vi "what.vi"() -> ()   [LabVIEW 2017]
uses:
  what.ctl
  <vilib>/myRIO/Instrument Drivers/Onboard IO/DIO/typedefs/DIO Reference.ctl
  <vilib>/myRIO/Common/Instrument Driver Framework/Utilities/typedefs/myRIO Generic Hardware Reference.ctl
  <vilib>/myRIO/Common/Instrument Driver Framework/Utilities/typedefs/Hardware Version Enum.ctl
  <vilib>/myRIO/Common/Instrument Driver Framework/Utilities/typedefs/myRIO v1.0 Reference.ctl
  <vilib>/myRIO/Common/Instrument Driver Framework/Utilities/typedefs/Generic FPGA Reference.ctl
  <vilib>/myRIO/Common/Instrument Driver Framework/myRIO v1.0/DIO/typedefs/DIO Channels List.ctl
  <vilib>/myRIO/Common/Instrument Driver Framework/myRIO v1.0/DIO/typedefs/DIO Channels Enum.ctl
  <vilib>/userdefined/High Color/nirio_resource_hc.ctl
  <vilib>/myRIO/Common/Instrument Driver Framework/Utilities/vis/Is FPGA Ref Available.vi
  <vilib>/myRIO/Common/Instrument Driver Framework/myRIO v1.0/DIO/vis/myRIO v1.1 Open DIO.vi
  <vilib>/myRIO/Instrument Drivers/Onboard IO/DIO/vis/Read.vi
  <vilib>/myRIO/Common/Instrument Driver Framework/Utilities/vis/Validate Channels.vi
  <vilib>/myRIO/Common/Instrument Driver Framework/myRIO v1.0/DIO/vis/myRIO v1.0 Reserve DIO.vi
  <vilib>/myRIO/Common/Instrument Driver Framework/myRIO v1.0/Resource Manager/vis/myRIO v1.0 Reserve Channel List.vi
  <vilib>/myRIO/Common/Instrument Driver Framework/myRIO v1.0/DIO/vis/myRIO v1.0 Build MUX Configuration DIO.vi
  <vilib>/myRIO/Common/Instrument Driver Framework/myRIO v1.0/Resource Manager/vis/myRIO v1.0 Reserve Channel.vi
  <vilib>/myRIO/Common/Instrument Driver Framework/myRIO v1.0/Resource Manager/vis/myRIO v1.0 Unreserve Channel.vi
  <vilib>/myRIO/Common/Instrument Driver Framework/myRIO v1.0/Resource Manager/vis/myRIO v1.0 Create Configuration List.vi
  <vilib>/myRIO/Common/Instrument Driver Framework/myRIO v1.0/Resource Manager/vis/myRIO v1.0 Build Mutex Name.vi
  <vilib>/Utility/VariantDataType/GetNumericInfo.vi
  <vilib>/Utility/error.llb/Error Cluster From Error Code.vi
  <vilib>/myRIO/Common/Instrument Driver Framework/myRIO v1.0/myRIO v1.1 Open.vi
  <vilib>/myRIO/Common/Instrument Driver Framework/Utilities/vis/IO Manager.vi
  <vilib>/myRIO/Common/Instrument Driver Framework/Utilities/vis/Configuration Manager.vi
  <vilib>/myRIO/Common/Instrument Driver Framework/myRIO v1.0/Resource Manager/vis/myRIO v1.0 Configure IO.vi
  <vilib>/myRIO/Common/Instrument Driver Framework/myRIO v1.0/myRIO v1.0 Close.vi
  <vilib>/myRIO/Common/Instrument Driver Framework/myRIO v1.0/DIO/vis/myRIO v1.0 Read DIO.vi
  <vilib>/myRIO/Express VI/Onboard IO/DI/DI Express VI.xnode
  <vilib>/myRIO/Instrument Drivers/Onboard IO/DIO/vis/myRIO DIO Open.xnode
  <vilib>/myRIO/Instrument Drivers/Onboard IO/DIO/DIO.lvlib
panel:
  out "index of element":i32
  in  "Abort":bool
  out "Counter Value":dbl
  in  "stop":bool
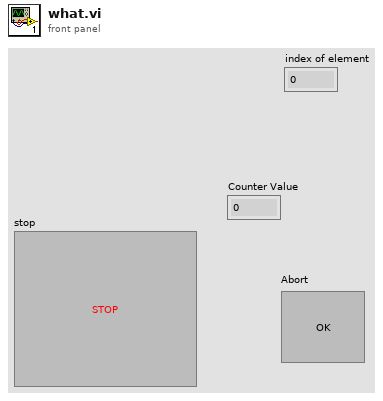
[diagram p1: front panel]
types:
  T1 = enum16{"off", "flash", "top", "middle", "bottom"}
  T2 = typedef "what.ctl" = enum16{"Initialize", "Floor 1", "Floor 2", "Floor 3", "GO!", "Stop!", "Wait for User Input"}
  T3 = typedef "DIO.lvlib/DIO Reference.ctl" = cluster{"myRIO Reference":T4, "DIO Channels List":T8}
  T4 = typedef "myRIO Generic Hardware Reference.ctl" = cluster{"myRIO Model":T5, "myRIO Hardware Reference":T6}
  T5 = typedef "Hardware Version Enum.ctl" = enum16{"Unknown", "myRIO-1900", "myRIO-1950", "roboRIO", "NI ELVIS RIO CM"}
  T6 = typedef "myRIO v1.0 Reference.ctl" = cluster{"Generic FPGA Reference":T7, "Allow multiple opens":bool}
  T7 = typedef "Generic FPGA Reference.ctl" = refnum<k20>
  T8 = typedef "DIO Channels List.ctl" = T9[]
  T9 = typedef "DIO Channels Enum.ctl" = enum16{"Not Connected", "C/DIO0", "C/DIO1", "C/DIO2", "C/DIO3", "C/DIO4", "C/DIO5", "C/DIO6", "C/DIO7", "A/DIO0", "A/DIO1", "A/DIO2", "A/DIO3", "A/DIO4", "A/DIO5", "A/DIO6", "A/DIO7", "A/DIO8", "A/DIO9", "A/DIO10", "A/DIO11", "A/DIO12", "A/DIO13", "A/DIO14", "A/DIO15", "B/DIO0", "B/DIO1", "B/DIO2", "B/DIO3", "B/DIO4", "B/DIO5", "B/DIO6", "B/DIO7", "B/DIO8", "B/DIO9", "B/DIO10", "B/DIO11", "B/DIO12", "B/DIO13", "B/DIO14", "B/DIO15", "LED0", "LED1", "LED2", "LED3", "Button0", "DIO/DIO0", "DIO/DIO1", "DIO/DIO2", "DIO/DIO3", "DIO/DIO4", "DIO/DIO5", "DIO/DIO6", "DIO/DIO7", "DIO/DIO8", "DIO/DIO9", "SPI/CS0", "SPI/CS1", "SPI/CS2", "SPI/CS3", "LED RADIO (Green)", "LED RADIO (Red)", "LED COMM (Green)", "LED COMM (Red)", "LED MODE (Green)", "LED MODE (Red)"}
  T10 = typedef "nirio_resource_hc.ctl" = tag
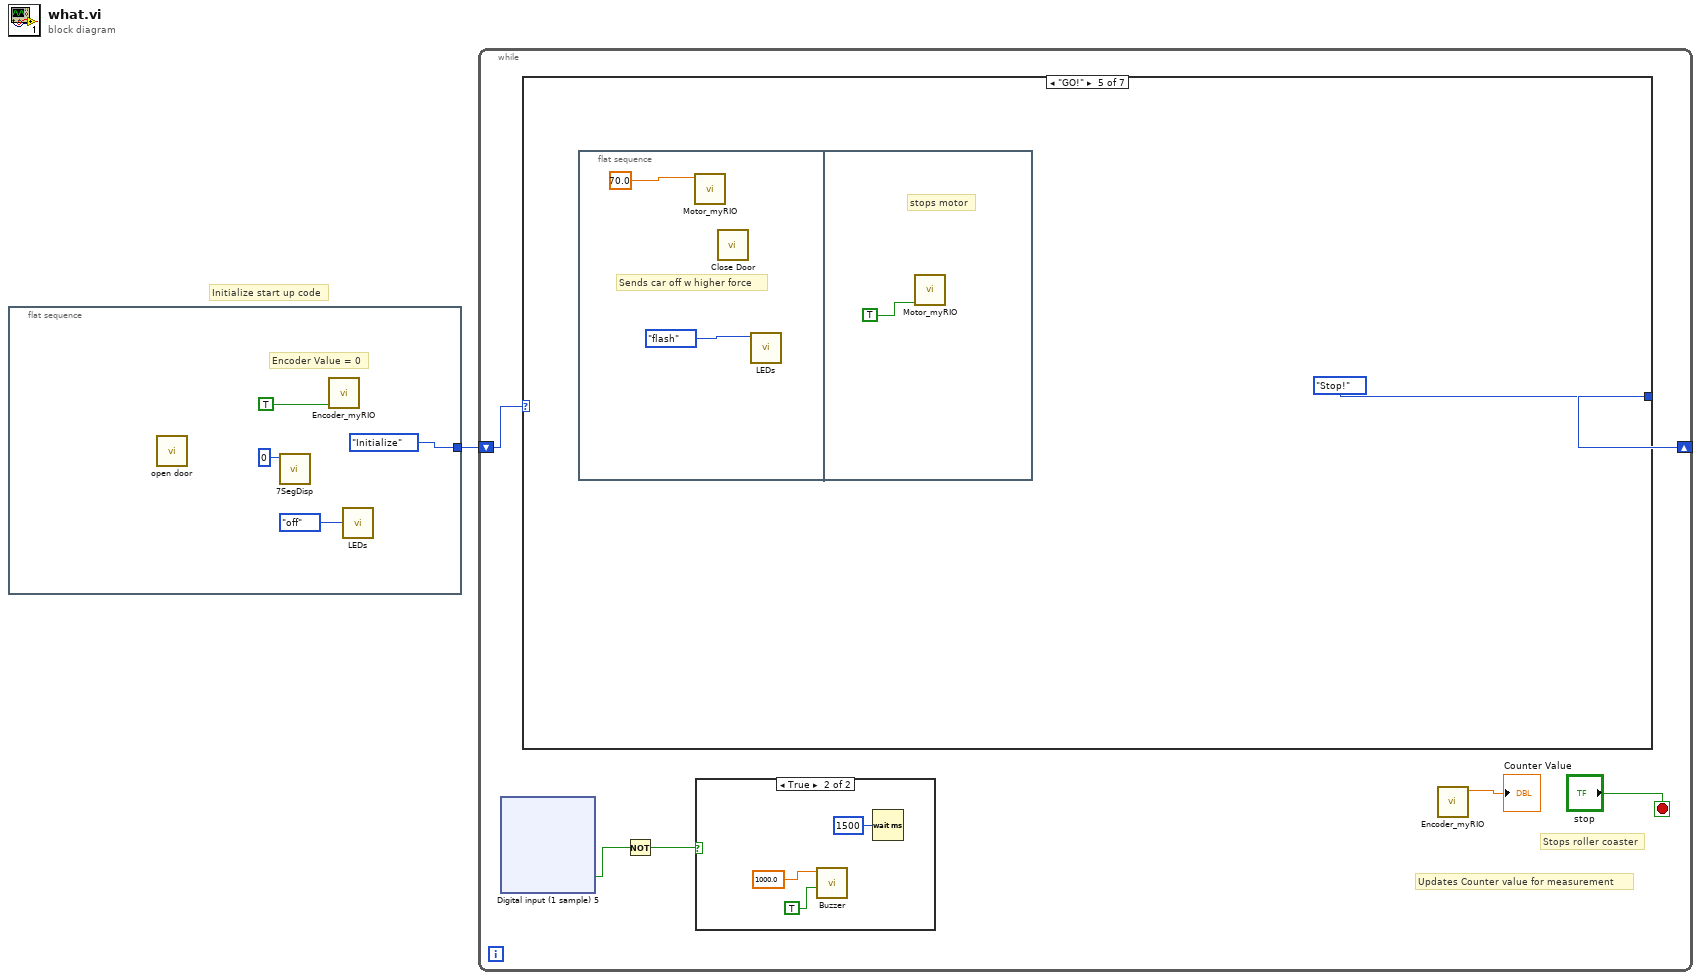
[diagram p0: block diagram]
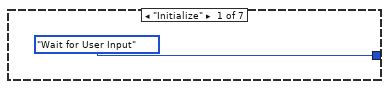
[diagram p3: hidden frame]
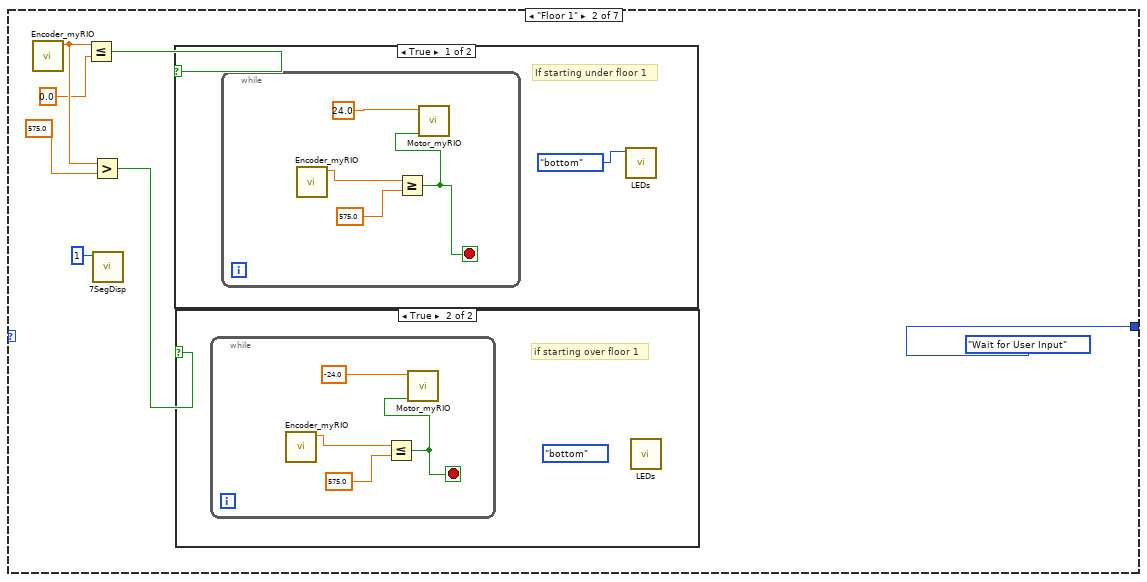
[diagram p4: hidden frame]
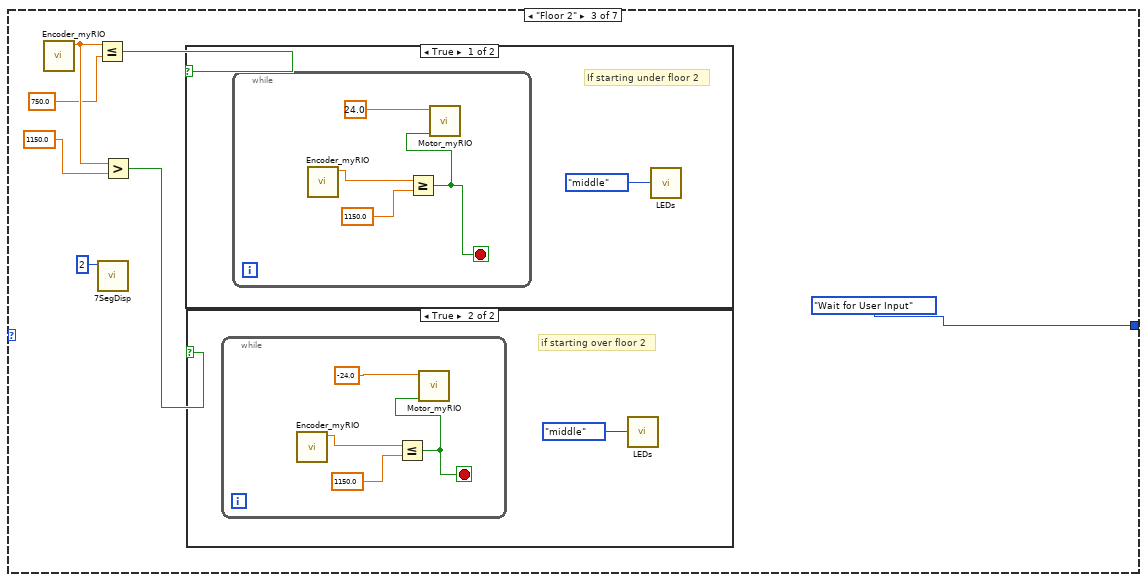
[diagram p7: hidden frame]
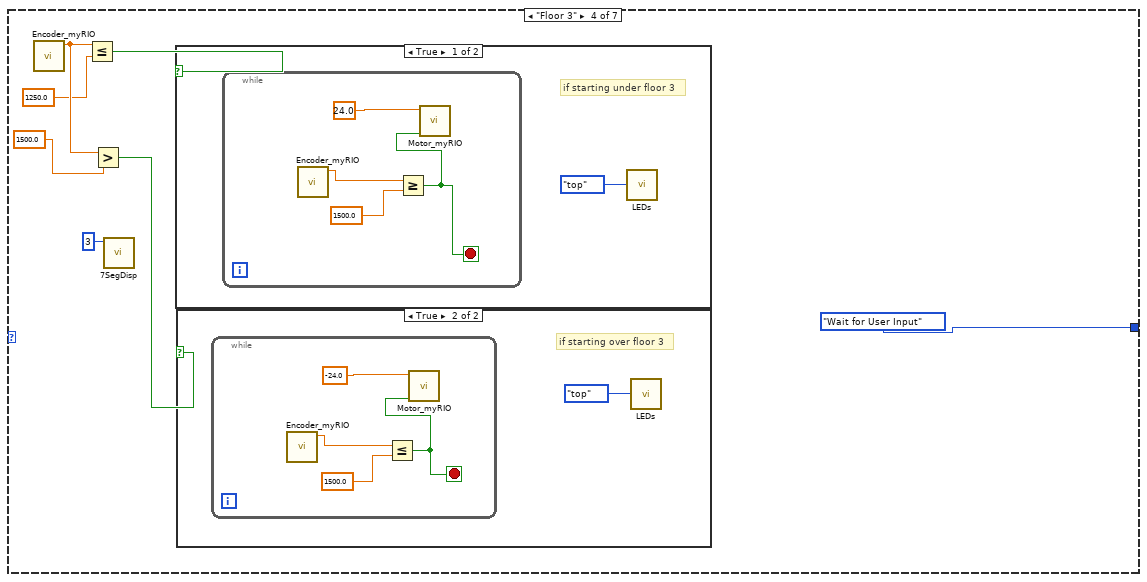
[diagram p10: hidden frame]
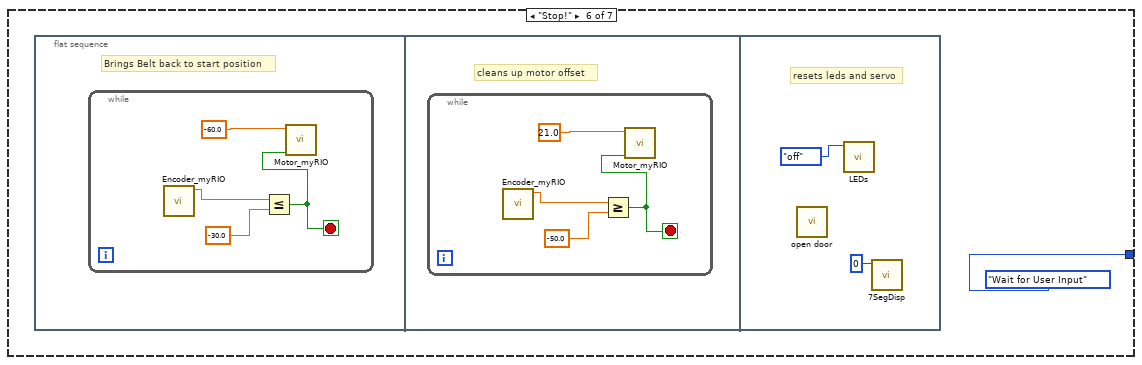
[diagram p13: hidden frame]
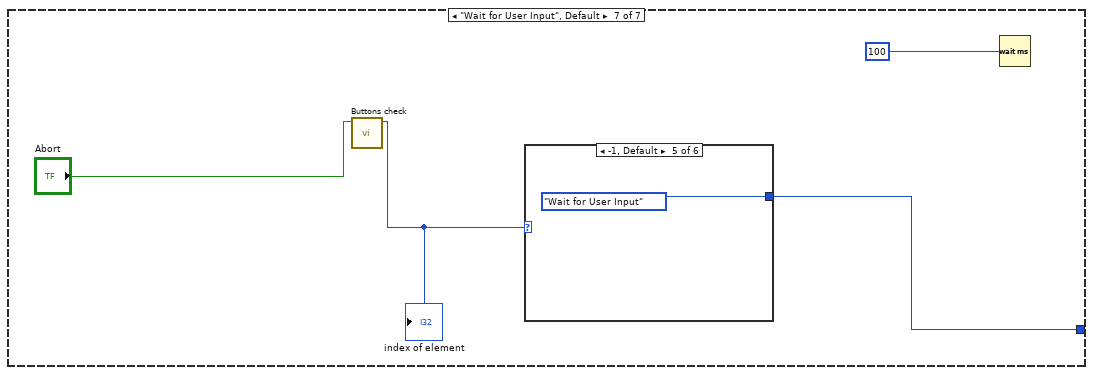
[diagram p14: hidden frame]
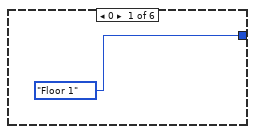
[diagram p15: hidden frame]
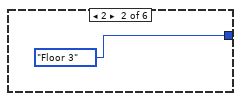
[diagram p16: hidden frame]
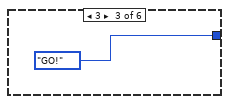
[diagram p17: hidden frame]
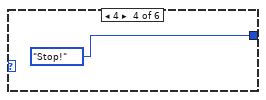
[diagram p18: hidden frame]
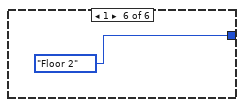
[diagram p19: hidden frame]
diagram:
  # "Initialize start up code"
  n1 = flat-sequence {
    tunnel: [what."Initialize"] -> w1
    frame #0 {
      # "Encoder Value = 0"
      n2 = call "open door.vi"() -> ()  [unwired: 12 in]
      n3 = call "7SegDisp.vi"("Input Number"=0) -> ()  [unwired: 11 in]
      n4 = call "Encoder_myRIO.vi"("Reset"=TRUE) -> ()  [unwired: 9 in, 2 out]
      n5 = call "LEDs.vi"("Enum"=T1."off") -> ()  [unwired: 11 in]
    }
  }
  n6 = while {
    shift-right: [w11] -> _
    shift-left: w1 -> [w8]
    stop <- "stop" stop-if-true
    # "Stops roller coaster"
    # "Updates Counter value for measurement"
    n7 = xnode "Digital input (1 sample) 5"() -> ("B/DIO14 (Pin 32)"=w6:bool)  [unwired: 1 in, 1 out]
    n8 = case shown="\"GO!\"" w8 {
      tunnel: [what."Wait for User Input" what."Wait for User Input" what."Wait for User Input" what."Wait for User Input" what."Stop!" what."Wait for User Input" w119] -> w11
      frame "Initialize" {
      }
      frame "Floor 1" {
        n9 = call "Encoder_myRIO.vi"() -> ("Counter Value"=w54:dbl)  [unwired: 10 in, 1 out]
        n10 = Less Or Equal?(x=w54, y=0.0) -> (x <= y?=w56:bool)
        n11 = Greater?(x=w54, y=575.0) -> (0:w55:bool)
        n12 = call "7SegDisp.vi"("Input Number"=1) -> ()  [unwired: 11 in]
        n13 = case shown="True" w56 {
          frame True {
            # "If starting under floor 1"
            n14 = while {
              stop <- w59 stop-if-true
              n15 = call "Encoder_myRIO.vi"() -> ("Counter Value"=w62:dbl)  [unwired: 10 in, 1 out]
              n16 = Greater Or Equal?(x=w62, y=575.0) -> (x >= y?=w59:bool)
              n17 = call "Motor_myRIO.vi"("Stop VI"=w59, "Duty Cycle (-100 to +100)"=24.0) -> ()  [unwired: 10 in]
            }
            n18 = call "LEDs.vi"("Enum"=T1."bottom") -> ()  [unwired: 11 in]
          }
          frame False {
          }
        }
        n19 = case shown="True" w55 {
          frame False {
          }
          frame True {
            (unwired) T1."bottom" ("Enum")
            # "if starting over floor 1"
            n20 = while {
              stop <- w63 stop-if-true
              n21 = call "Encoder_myRIO.vi"() -> ("Counter Value"=w66:dbl)  [unwired: 10 in, 1 out]
              n22 = Less Or Equal?(x=w66, y=575.0) -> (x <= y?=w63:bool)
              n23 = call "Motor_myRIO.vi"("Stop VI"=w63, "Duty Cycle (-100 to +100)"=-24.0) -> ()  [unwired: 10 in]
            }
            n24 = call "LEDs.vi"() -> ()  [unwired: 12 in]
          }
        }
      }
      frame "Floor 2" {
        n25 = call "Encoder_myRIO.vi"() -> ("Counter Value"=w70:dbl)  [unwired: 10 in, 1 out]
        n26 = Less Or Equal?(x=w70, y=750.0) -> (x <= y?=w72:bool)
        n27 = call "7SegDisp.vi"("Input Number"=2) -> ()  [unwired: 11 in]
        n28 = Greater?(x=w70, y=1150.0) -> (0:w71:bool)
        n29 = case shown="True" w72 {
          frame True {
            # "If starting under floor 2"
            n30 = while {
              stop <- w75 stop-if-true
              n31 = call "Encoder_myRIO.vi"() -> ("Counter Value"=w78:dbl)  [unwired: 10 in, 1 out]
              n32 = Greater Or Equal?(x=w78, y=1150.0) -> (x >= y?=w75:bool)
              n33 = call "Motor_myRIO.vi"("Stop VI"=w75, "Duty Cycle (-100 to +100)"=24.0) -> ()  [unwired: 10 in]
            }
            n34 = call "LEDs.vi"("Enum"=T1."middle") -> ()  [unwired: 11 in]
          }
          frame False {
          }
        }
        n35 = case shown="True" w71 {
          frame False {
          }
          frame True {
            # "if starting over floor 2"
            n36 = while {
              stop <- w80 stop-if-true
              n37 = call "Encoder_myRIO.vi"() -> ("Counter Value"=w83:dbl)  [unwired: 10 in, 1 out]
              n38 = Less Or Equal?(x=w83, y=1150.0) -> (x <= y?=w80:bool)
              n39 = call "Motor_myRIO.vi"("Stop VI"=w80, "Duty Cycle (-100 to +100)"=-24.0) -> ()  [unwired: 10 in]
            }
            n40 = call "LEDs.vi"("Enum"=T1."middle") -> ()  [unwired: 11 in]
          }
        }
      }
      frame "Floor 3" {
        n41 = call "Encoder_myRIO.vi"() -> ("Counter Value"=w87:dbl)  [unwired: 10 in, 1 out]
        n42 = Less Or Equal?(x=w87, y=1250.0) -> (x <= y?=w89:bool)
        n43 = Greater?(x=w87, y=1500.0) -> (0:w88:bool)
        n44 = call "7SegDisp.vi"("Input Number"=3) -> ()  [unwired: 11 in]
        n45 = case shown="True" w89 {
          frame True {
            # "if starting under floor 3"
            n46 = while {
              stop <- w92 stop-if-true
              n47 = call "Encoder_myRIO.vi"() -> ("Counter Value"=w95:dbl)  [unwired: 10 in, 1 out]
              n48 = Greater Or Equal?(x=w95, y=1500.0) -> (x >= y?=w92:bool)
              n49 = call "Motor_myRIO.vi"("Stop VI"=w92, "Duty Cycle (-100 to +100)"=24.0) -> ()  [unwired: 10 in]
            }
            n50 = call "LEDs.vi"("Enum"=T1."top") -> ()  [unwired: 11 in]
          }
          frame False {
          }
        }
        n51 = case shown="True" w88 {
          frame False {
          }
          frame True {
            # "if starting over floor 3"
            n52 = while {
              stop <- w98 stop-if-true
              n53 = call "Encoder_myRIO.vi"() -> ("Counter Value"=w100:dbl)  [unwired: 10 in, 1 out]
              n54 = Less Or Equal?(x=w100, y=1500.0) -> (x <= y?=w98:bool)
              n55 = call "Motor_myRIO.vi"("Stop VI"=w98, "Duty Cycle (-100 to +100)"=-24.0) -> ()  [unwired: 10 in]
            }
            n56 = call "LEDs.vi"("Enum"=T1."top") -> ()  [unwired: 11 in]
          }
        }
      }
      frame "GO!" {
        n57 = flat-sequence {
          frame #0 {
            # "Sends car off w higher force"
            n58 = call "Motor_myRIO.vi"("Duty Cycle (-100 to +100)"=70.0) -> ()  [unwired: 11 in]
            n59 = call "Close Door.vi"() -> ()  [unwired: 12 in]
            n60 = call "LEDs.vi"("Enum"=T1."flash") -> ()  [unwired: 11 in]
          }
          frame #1 {
            # "stops motor"
            n61 = call "Motor_myRIO.vi"("Stop VI"=TRUE) -> ()  [unwired: 11 in]
          }
        }
      }
      frame "Stop!" {
        n62 = flat-sequence {
          frame #0 {
            # "Brings Belt back to start position"
            n63 = while {
              stop <- w106 stop-if-true
              n64 = call "Encoder_myRIO.vi"() -> ("Counter Value"=w109:dbl)  [unwired: 10 in, 1 out]
              n65 = Less Or Equal?(x=w109, y=-30.0) -> (x <= y?=w106:bool)
              n66 = call "Motor_myRIO.vi"("Stop VI"=w106, "Duty Cycle (-100 to +100)"=-60.0) -> ()  [unwired: 10 in]
            }
          }
          frame #1 {
            # "cleans up motor offset"
            n67 = while {
              stop <- w110 stop-if-true
              n68 = call "Encoder_myRIO.vi"() -> ("Counter Value"=w113:dbl)  [unwired: 10 in, 1 out]
              n69 = Greater Or Equal?(x=w113, y=-50.0) -> (x >= y?=w110:bool)
              n70 = call "Motor_myRIO.vi"("Stop VI"=w110, "Duty Cycle (-100 to +100)"=21.0) -> ()  [unwired: 10 in]
            }
          }
          frame #2 {
            # "resets leds and servo"
            n71 = call "open door.vi"() -> ()  [unwired: 12 in]
            n72 = call "LEDs.vi"("Enum"=T1."off") -> ()  [unwired: 11 in]
            n73 = call "7SegDisp.vi"("Input Number"=0) -> ()  [unwired: 11 in]
          }
        }
      }
      frame "Wait for User Input", Default {
        n74 = call "Buttons check.vi"("Abort"="Abort") -> ("index of element"=w117:i32)  [unwired: 10 in]
        "index of element" <- w117
        n75 = case shown="-1, Default" w117 {
          tunnel: [what."Floor 1" what."Floor 3" what."GO!" what."Stop!" what."Wait for User Input" what."Floor 2"] -> w119
          frame 0 {
          }
          frame 2 {
          }
          frame 3 {
          }
          frame 4 {
          }
          frame -1, Default {
          }
          frame 1 {
          }
        }
        n76 = Wait (ms)(milliseconds to wait=u32 100) -> ()  [unwired: 1 out]
      }
    }
    n77 = Not(x=w6) -> (.not. x?=w7:bool)
    n78 = case shown="True" w7 {
      frame False {
      }
      frame True {
        n79 = call "Buzzer.vi"("stop"=TRUE, "frequency [Hz]"=1000.0) -> ()  [unwired: 10 in]
        n80 = Wait (ms)(milliseconds to wait=u32 1500) -> ()  [unwired: 1 out]
      }
    }
    n81 = call "Encoder_myRIO.vi"() -> ("Counter Value"=→"Counter Value":dbl)  [unwired: 10 in, 1 out]
  }
